vi "Page_Advanced_Initialize.vi"(6 "ctl references":T1, 8 "error in (no error)":errorcluster, 11 "AB_SourceDistribution in":refnum<class "AB_SourceDistribution.lvclass">) -> (0 "error out":errorcluster, 3 "AB_SourceDistribution out":refnum<class "AB_SourceDistribution.lvclass">)   [LabVIEW 2020, in "AB_SourceDistribution.lvclass"]
uses:
  <vilib>/AppBuilder/AB_Classes/SourceDistribution/AB_SourceDistribution.lvclass
  <resource>/Framework/Providers/Builds/AppBuilder/AB_UI_Page_Advanced_References.ctl
  <vilib>/AppBuilder/AB_Classes/Build/AB_Build.lvclass
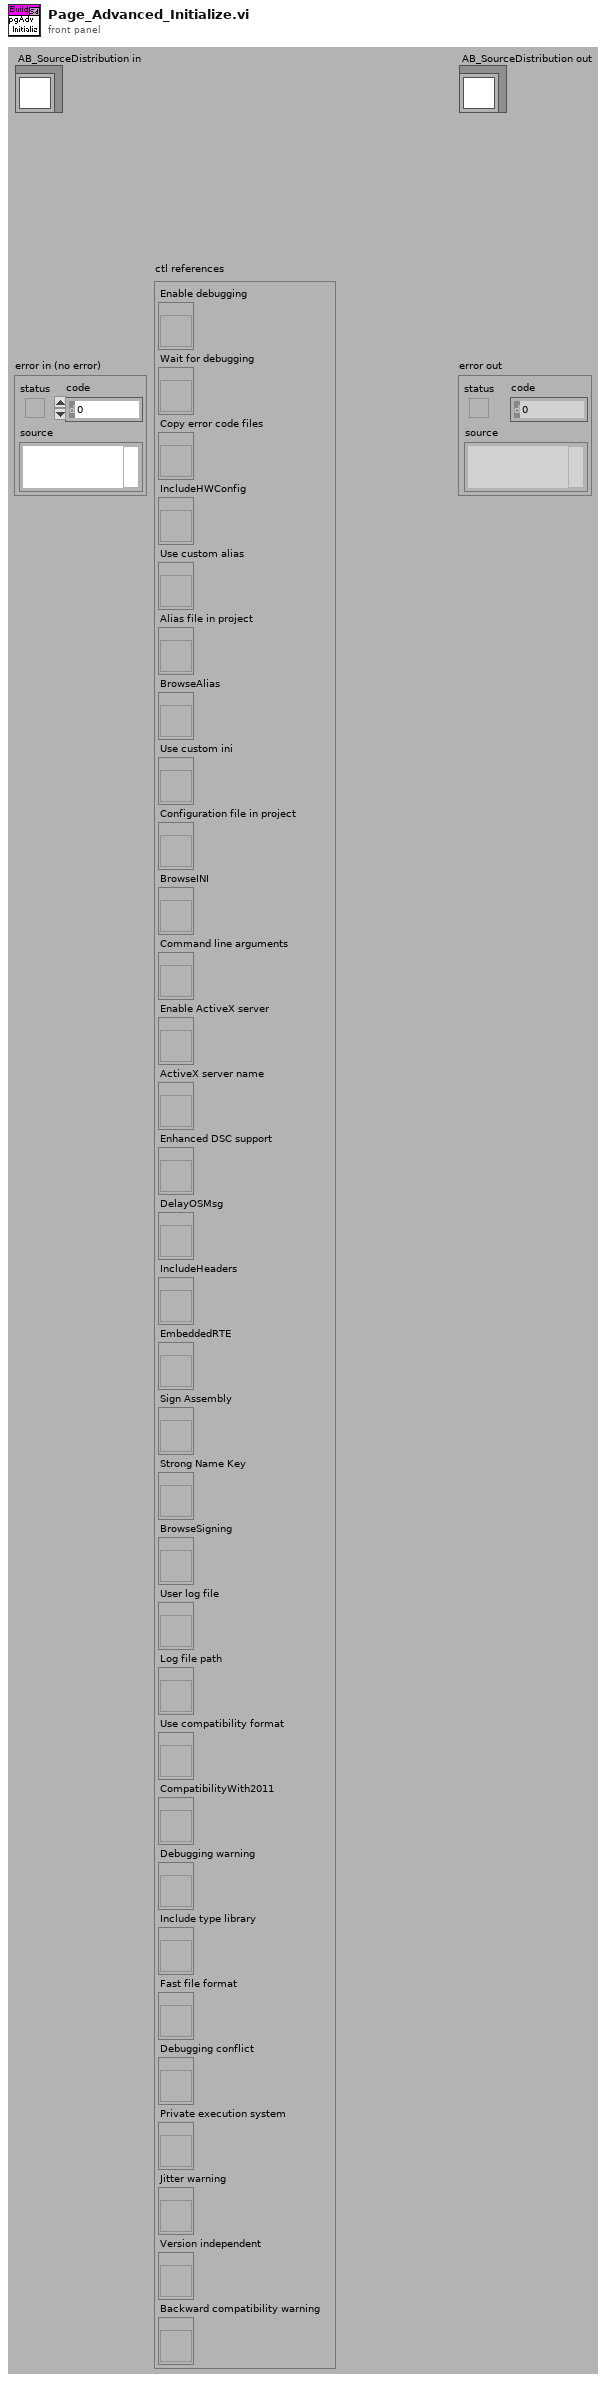
[diagram p1: front panel]
types:
  T1 = typedef "AB_UI_Page_Advanced_References.ctl" = cluster{"Enable debugging":refnum<vi>, "Wait for debugging":refnum<vi>, "Copy error code files":refnum<vi>, "IncludeHWConfig":refnum<vi>, "Use custom alias":refnum<vi>, "Alias file in project":refnum<vi>, "BrowseAlias":refnum<vi>, "Use custom ini":refnum<vi>, "Configuration file in project":refnum<vi>, "BrowseINI":refnum<vi>, "Command line arguments":refnum<vi>, "Enable ActiveX server":refnum<vi>, "ActiveX server name":refnum<vi>, "Enhanced DSC support":refnum<vi>, "DelayOSMsg":refnum<vi>, "IncludeHeaders":refnum<vi>, "EmbeddedRTE":refnum<vi>, "Sign Assembly":refnum<vi>, "Strong Name Key":refnum<vi>, "BrowseSigning":refnum<vi>, "User log file":refnum<vi>, "Log file path":refnum<vi>, "Use compatibility format":refnum<vi>, "CompatibilityWith2011":refnum<vi>, "Debugging warning":refnum<vi>, "Include type library":refnum<vi>, "Fast file format":refnum<vi>, "Debugging conflict":refnum<vi>, "Private execution system":refnum<vi>, "Jitter warning":refnum<vi>, "Version independent":refnum<vi>, "Backward compatibility warning":refnum<vi>}
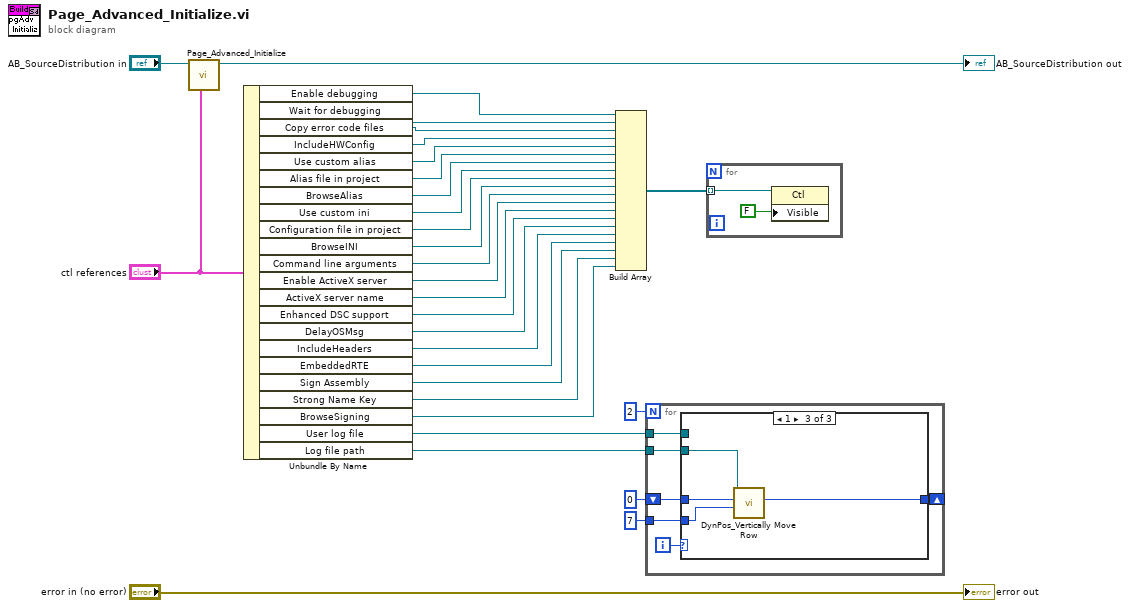
[diagram p0: block diagram]
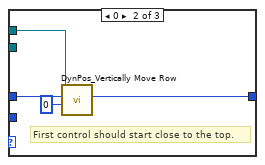
[diagram p3: hidden frame]
diagram:
  n1 = call-parent "Page_Advanced_Initialize.vi"("ctl references"="ctl references", "AB_Build in"="AB_SourceDistribution in") -> ("AB_Build out"=→"AB_SourceDistribution out":refnum<class "AB_SourceDistribution.lvclass">)  [unwired: 1 in, 8 out]
  n2 = Unbundle By Name("ctl references") -> ("Enable debugging"=w26:refnum<vi>, "Wait for debugging"=w25:refnum<vi>, "Copy error code files"=w24:refnum<vi>, "IncludeHWConfig"=w23:refnum<vi>, "Use custom alias"=w22:refnum<vi>, "Alias file in project"=w21:refnum<vi>, "BrowseAlias"=w20:refnum<vi>, "Use custom ini"=w19:refnum<vi>, "Configuration file in project"=w18:refnum<vi>, "BrowseINI"=w17:refnum<vi>, "Command line arguments"=w16:refnum<vi>, "Enable ActiveX server"=w15:refnum<vi>, "ActiveX server name"=w14:refnum<vi>, "Enhanced DSC support"=w13:refnum<vi>, "DelayOSMsg"=w11:refnum<vi>, "IncludeHeaders"=w10:refnum<vi>, "EmbeddedRTE"=w9:refnum<vi>, "Sign Assembly"=w8:refnum<vi>, "Strong Name Key"=w7:refnum<vi>, "BrowseSigning"=w6:refnum<vi>, "User log file"=w4:refnum<vi>, "Log file path"=w3:refnum<vi>)
  n3 = Build Array(w26, w25, w24, w23, w22, w21, w20, w19, w18, w17, w16, w15, w14, w13, w11, w10, w9, w8, w7, w6) -> (w12:refnum<vi>[])
  n4 = for {
    N: 2 -> [_]
    tunnel: w4 -> [w35]
    tunnel: w3 -> [w34]
    shift-right: [w33] -> _
    shift-left: 0 ("Bottom pixel") -> [w32]
    tunnel: 7 ("Bottom pixel") -> [w31]
    i -> [w36]
    n5 = case shown="1" w36 {
      tunnel: w35 -> [_ w40 _]
      tunnel: w34 -> [_ _ w42]
      tunnel: [w37 w39 w45] -> w33
      tunnel: w32 -> [w37 w38 w44]
      tunnel: w31 -> [_ _ w43]
      frame Default {
      }
      frame 0 {
        # "First control should start close to the top."
        n6 = call <vilib>:"DynPos_Vertically Move Row.vi"("Pixel separation (6)"=0, "Bottom of last control"=w38, "Control"=w40) -> ("Bottom pixel"=w39:i32)  [unwired: 1 in, 7 out]
      }
      frame 1 {
        n7 = call <vilib>:"DynPos_Vertically Move Row.vi"("Pixel separation (6)"=w43, "Bottom of last control"=w44, "Control"=w42) -> ("Bottom pixel"=w45:i32)  [unwired: 1 in, 7 out]
      }
    }
  }
  n8 = for {
    tunnel: w12 -> [w47] mode=indexing
    n9 = property class="Ctl"(reference=w47, "Visible"=FALSE) -> ()  [unwired: 1 in, 2 out]
  }
  "error out" <- "error in (no error)"
